vi "Add Password.vi"(8 "error in (no error)":errorcluster, 10 "Write Password":string, 11 "Masterv2 in":refnum<class "Masterv2.lvclass">) -> (0 "error out":errorcluster, 3 "Masterv2 out":refnum<class "Masterv2.lvclass">)   [LabVIEW 2014, in "Main Libraryv2.lvlib" / "Masterv2.lvclass"]
uses:
  Master/Masterv2.lvclass
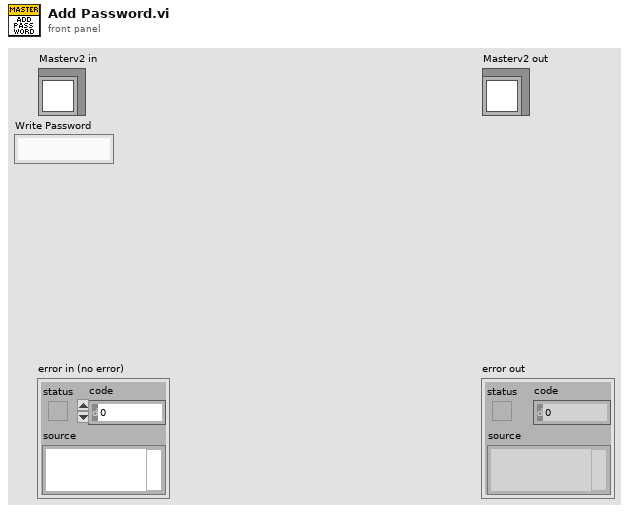
[diagram p1: front panel]
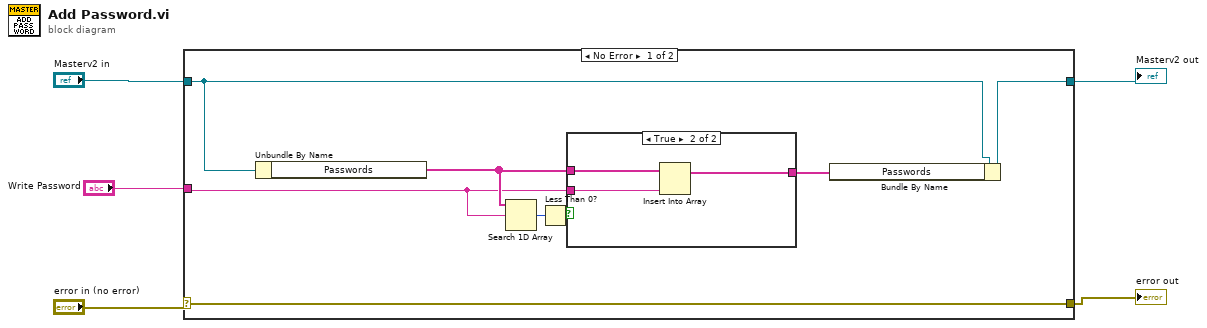
[diagram p0: block diagram]
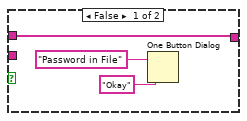
[diagram p2: hidden frame]
diagram:
  n1 = case shown="No Error" "error in (no error)" {
    selector: "error in (no error)" -> [w13 w21]
    tunnel: [w13 w21] -> w4
    tunnel: [w7 w20] -> w2
    tunnel: "Masterv2 in" -> [w8 w20]
    tunnel: "Write Password" -> [w6 _]
    frame No Error {
      n2 = Unbundle By Name(w8) -> ("Passwords"=w11:string[])
      n3 = Search 1D Array(1D array=w11, element=w6) -> (index of element=w10:i32)  [unwired: 1 in]
      n4 = Less Than 0?(x=w10) -> (x < 0?=w9:bool)
      n5 = case shown="True" w9 {
        tunnel: [w16 w19] -> w12
        tunnel: w11 -> [w16 w18]
        tunnel: w6 -> [_ w17]
        frame False {
          n6 = One Button Dialog(message="Password in File", button name ("OK")="Okay") -> ()  [unwired: 1 out]
        }
        frame True {
          n7 = Insert Into Array(array=w18, new element=w17) -> (w19:string[])  [unwired: 1 in]
        }
      }
      n8 = Bundle By Name(cluster=w8, "Passwords"=w12) -> (w7:refnum<class "Masterv2.lvclass">)
    }
    frame Error {
    }
  }
  "error out" <- w4
  "Masterv2 out" <- w2
